vi "Get_AppData_Path.vi"() -> (0 "path":path)   [LabVIEW 2018]
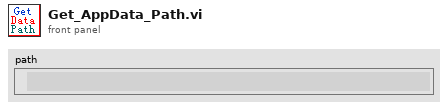
[diagram p1: front panel]
types:
  T1 = enum32{"invalid app kind", "Development System", "Run Time System", "Student Edition", "Embedded LabVIEW", "Evaluation", "Custom"}
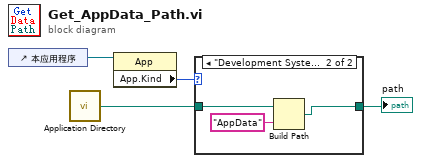
[diagram p0: block diagram]
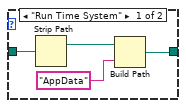
[diagram p2: hidden frame]
diagram:
  n1 = control-ref of="本应用程序"() -> (w4:refnum<vi>)
  n2 = call <vilib>:"Application Directory.vi"() -> ("Application Directory"=w1:path)
  n3 = property class="App"(reference=w4) -> ("App.Kind"=w3:T1)  [unwired: 1 in, 2 out]
  n4 = case shown="\"Development System\", 默认" w3 {
    tunnel: w1 -> [w8 w11]
    tunnel: [w7 w9] -> w2
    frame "Run Time System" {
      n5 = Strip Path(path=w8) -> (stripped path=w6:path)  [unwired: 1 out]
      n6 = Build Path(base path=w6, name or relative path="AppData" ("名称或相对路径")) -> (appended path=w7:path)
    }
    frame "Development System", Default {
      n7 = Build Path(base path=w11, name or relative path="AppData" ("名称或相对路径")) -> (appended path=w9:path)
    }
  }
  "path" <- w2
